vi "Do This.vi"(8 "error in (no error)":errorcluster, 10 "Status Events":refnum<class "Status Events.lvclass">, 11 "VIP Publish in":refnum<class "VIP Publish.lvclass">) -> (0 "error out":errorcluster, 3 "VIP Publish out":refnum<class "VIP Publish.lvclass">)   [LabVIEW 2014, in "VIP Publish.lvclass"]
uses:
  VIP Publish.lvclass
  Shared/Classes/Status Events/Status Events.lvclass
  VIP Publish.lvclass/VIP Publish.ctl
  <vilib>/Utility/error.llb/DialogType.ctl
  Classes/Job/Job.lvclass/Job.ctl
  Classes/Job/Job.lvclass
  <vilib>/JKI/VIPM API/VIPM API_vipm_api.lvlib
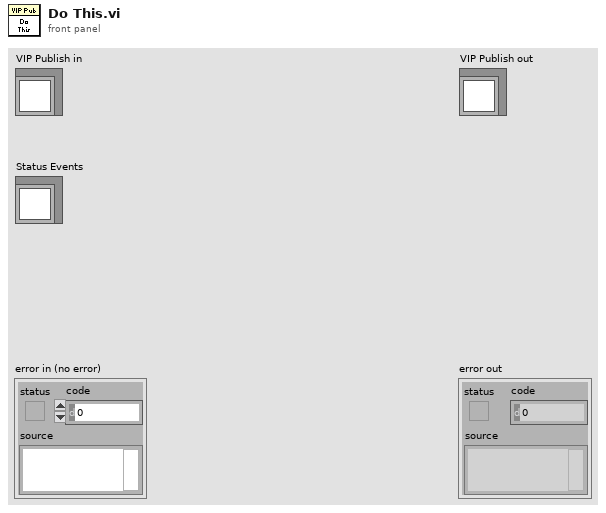
[diagram p1: front panel]
types:
  T1 = typedef "DialogType.ctl" = u16
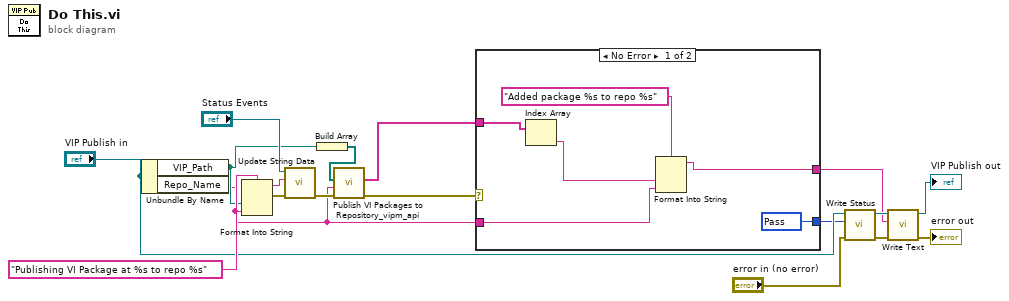
[diagram p0: block diagram]
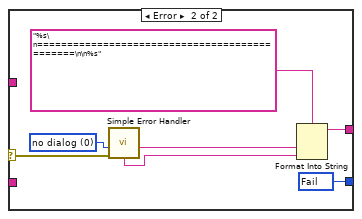
[diagram p2: hidden frame]
diagram:
  n1 = Unbundle By Name("VIP Publish in") -> ("VIP_Path"=w3:path, "Repo_Name"=w1:string)
  n2 = Format Into String(format string="Publishing VI Package at %s to repo %s", w3, w1) -> (resulting string=w17:string, error out=w9:errorcluster)  [unwired: 2 in]
  n3 = call "Update String Data.vi"("error in (no error)"=w9, "String Data"=w17, "Status Updater in"="Status Events") -> ("error out"=w5:errorcluster)  [unwired: 7 in, 1 out]
  n4 = Build Array(w3) -> (w2:path[])
  n5 = call <vilib>:"Publish VI Packages to Repository_vipm_api.vi"("error in (no error)"=w5, "Repository Name"=w1, "Packages to publish to Repository Library (vip,ogp)"=w2) -> ("error out"=w8:errorcluster, "Package Names Published"=w4:string[])  [unwired: 7 in]
  n6 = case shown="No Error" w8 {
    selector: w8 -> [_ w30]
    tunnel: [w24 w31] -> w11
    tunnel: [w19 w25] -> w12
    tunnel: w4 -> [w23 _]
    tunnel: w1 -> [w20 _]
    frame No Error {
      w24 = u16 200 items=["Abort"=503, "Fail"=500, "Pass"=200] ("Status")
      n7 = Index Array(array=w23) -> (element=w21:string)  [unwired: 1 in]
      n8 = Format Into String(format string="Added package %s to repo %s", w21, w20) -> (resulting string=w19:string)  [unwired: 2 in, 1 out]
    }
    frame Error {
      w29 = T1 0 items=["no dialog", "OK message", "continue or stop message", "OK message + warnings", "continue/stop + warnings"] ("type of dialog (OK msg:1)")
      w31 = u16 500 items=["Abort"=503, "Fail"=500, "Pass"=200] ("Status")
      n9 = call <vilib>:"Simple Error Handler.vi"("type of dialog (OK msg:1)"=w29, "error in (no error)"=w30) -> ("source out"=w27:string, "message"=w26:string)  [unwired: 3 in, 3 out]
      n10 = Format Into String(format string="%s\n==============================================\n\n%s", w27, w26) -> (resulting string=w25:string)  [unwired: 2 in, 1 out]
    }
  }
  n11 = call "Write Status.vi"("error in (no error)"="error in (no error)", "Status"=w11, "Job in"="VIP Publish in") -> ("error out"=w13:errorcluster, "Job out"=w14:refnum<class "VIP Publish.lvclass">)  [unwired: 7 in]
  n12 = call "Write Text.vi"("error in (no error)"=w13, "Text"=w12, "Job in"=w14) -> ("error out"=→"error out":errorcluster, "Job out"=→"VIP Publish out":refnum<class "VIP Publish.lvclass">)  [unwired: 7 in]
